vi "DateTimeToIntegerDateTime.vi"(10 "Datetime string":string) -> (1 "Time":i32, 3 "Date":i32)   [LabVIEW 2012]
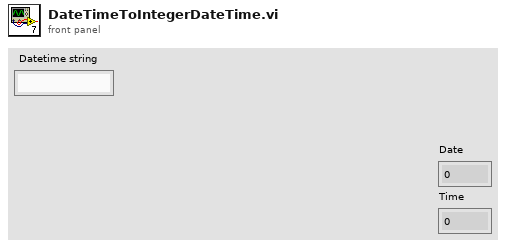
[diagram p1: front panel]
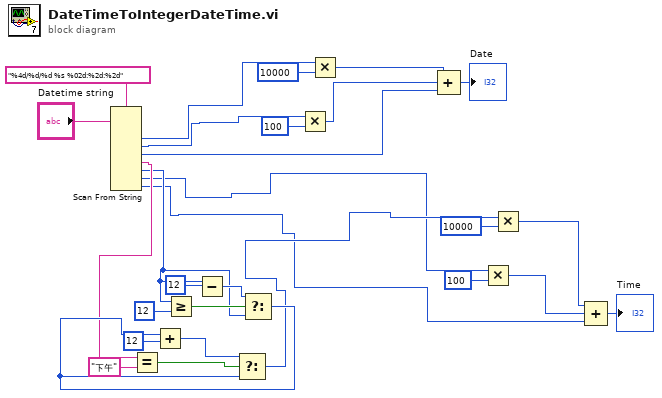
[diagram p0: block diagram]
diagram:
  n1 = Scan From String(format string="%4d/%d/%d %s %02d:%2d:%2d", input string="Datetime string") -> (output 1=w16:i32, output 2=w14:i32, output 3=w10:i32, output 4=w19:string, output 5=w18:i32, output 6=w6:i32, output 7=w3:i32)  [unwired: 9 in, 3 out]
  n2 = Equal?(x=w19, y="下午") -> (x = y?=w24:bool)
  n3 = Greater Or Equal?(x=w18, y=12) -> (x >= y?=w28:bool)
  n4 = Subtract(x=w18, y=12) -> (x-y=w26:i32)
  n5 = Select(t=w26, s=w28, f=w18) -> (s? t:f=w20:i32)
  n6 = Add(x=w20, y=12) -> (x+y=w21:i32)
  n7 = Select(t=w21, s=w24, f=w20) -> (s? t:f=w7:i32)
  n8 = Multiply(x=w14, y=100) -> (x*y=w11:i32)
  n9 = Multiply(x=w16, y=10000) -> (x*y=w12:i32)
  n10 = Compound Arithmetic op=ADD(w12, w11, w10) -> (→"Date":i32)
  n11 = Multiply(x=w6, y=100) -> (x*y=w4:i32)
  n12 = Multiply(x=w7, y=10000) -> (x*y=w5:i32)
  n13 = Compound Arithmetic op=ADD(w5, w4, w3) -> (→"Time":i32)
